vi "OPCServerSettings.vi"() -> (0 "OK Button 2":bool)   [LabVIEW 2025]
uses:
  <vilib>/Utility/config.llb/NI_LVConfig.lvlib
  <vilib>/Utility/config.llb/Read Key (String).vi
  <vilib>/Utility/config.llb/Write Key (String).vi
panel:
  in  "Cancel Button":bool
  in  "OK Button":bool
  in  "OPC Server Address":string
  # "OPC Server Settings"
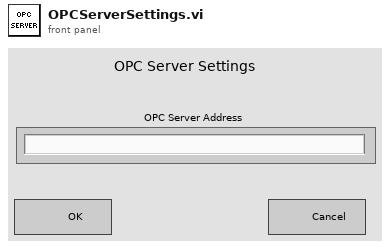
[diagram p1: front panel]
types:
  T1 = typedef "NI_LVConfig.lvlib/Config Data RefNum.ctl" = refnum<k1>
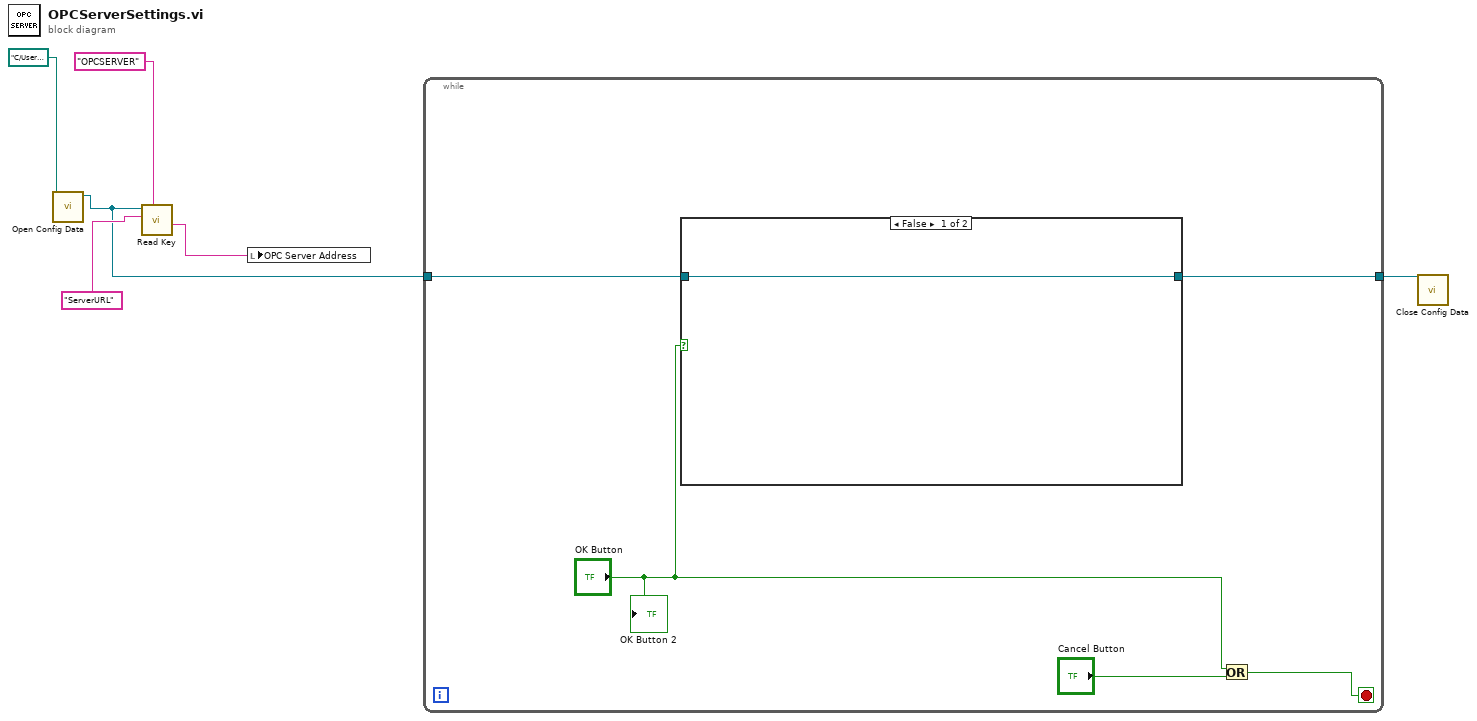
[diagram p0: block diagram]
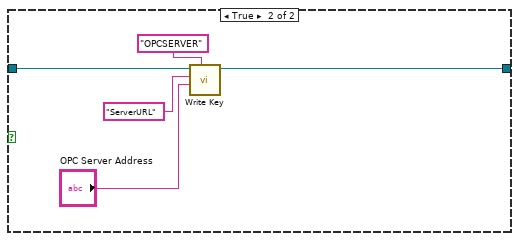
[diagram p2: hidden frame]
diagram:
  n1 = call <vilib>:"Open Config Data.vi"("configuration file path"=path "C:/Users/magne/OneDrive/Dokumenter/Skole/IIA2017-1 26V Industrial Information Technology/Assignments/SCADA Assignment/02 Files/Task 3/settings.ini") -> ("refnum"=w2:T1)  [unwired: 8 in, 2 out]
  n2 = call-poly <vilib>:"Read Key.vi"("section"="OPCSERVER", "key"="ServerURL", "refnum"=w2) -> ("value"=w3:string)  [unwired: 5 in, 3 out]
  n3 = local write "OPC Server Address"(w3) -> ()
  n4 = while {
    tunnel: w2 -> [w9]
    tunnel: [w8] -> w1
    stop <- w10 stop-if-true
    n5 = case shown="False" "OK Button" {
      tunnel: w9 -> [w12 w17]
      tunnel: [w12 w13] -> w8
      frame False {
      }
      frame True {
        n6 = call-poly <vilib>:"Write Key.vi"("section"="OPCSERVER", "value"="OPC Server Address", "key"="ServerURL", "refnum"=w17) -> ("refnum out"=w13:T1)  [unwired: 5 in, 2 out]
      }
    }
    n7 = Or(x="OK Button", y="Cancel Button") -> (x .or. y?=w10:bool)
    "OK Button 2" <- "OK Button"
  }
  n8 = call <vilib>:"Close Config Data.vi"("refnum"=w1) -> ()  [unwired: 9 in, 2 out]
